vi "Spatial Dual Decode Packet 20 (SubVI).vi"(0 "Packet 20 Bytes In":u8[](array[numeric]), 9 "String Precision":i16) -> (2 "Packet 20 Decoded Data Cluster":T1, 4 "Channel Names":string[](array[string])=["Unix TS", "uS", "Latitude", "Longitude", "Height (m)", "Vel N (m/s)", "Vel E (m/s)", "Vel D (m/s)", "G force (g)", "Pitch (deg)", "Roll (deg)", "Heading (deg)", "Body Acc X (m/s/s)", "Body Acc Y (m/s/s)", "Body Acc Z (m/s/s)", "Angular Vel X (rad/s)", "Angular Vel Y (rad/s)", "Angular Vel Z (rad/s)"], 6 "Data":string[](array[string]), 10 "Channel Units":string[](array[string])=["Unix TS", "uS", "Latitude", "Longitude", "Height (m)", "Vel N (m/s)", "Vel E (m/s)", "Vel D (m/s)", "G force (g)", "Pitch (deg)", "Roll (deg)", "Heading (deg)", "Body Acc X (m/s/s)", "Body Acc Y (m/s/s)", "Body Acc Z (m/s/s)", "Angular Vel X (rad/s)", "Angular Vel Y (rad/s)", "Angular Vel Z (rad/s)"], 14 "Unix Timestamp":u64, 15 "Data Types":string[](array[string])=["seconds", "uS", "deg", "deg", "m", "m/s", "m/s", "m/s", "g", "deg", "deg", "deg", "m/s/s", "m/s/s", "m/s/s", "rad/sec", "rad/sec", "rad/sec"])   [LabVIEW 2019, in "SpatialDual_Parsers.lvlib"]
uses:
  SpatialDual_Parsers.lvlib
  Globals and Definitions/RT Globals RD v1.0.vi
panel:
  out "uS Period":u32
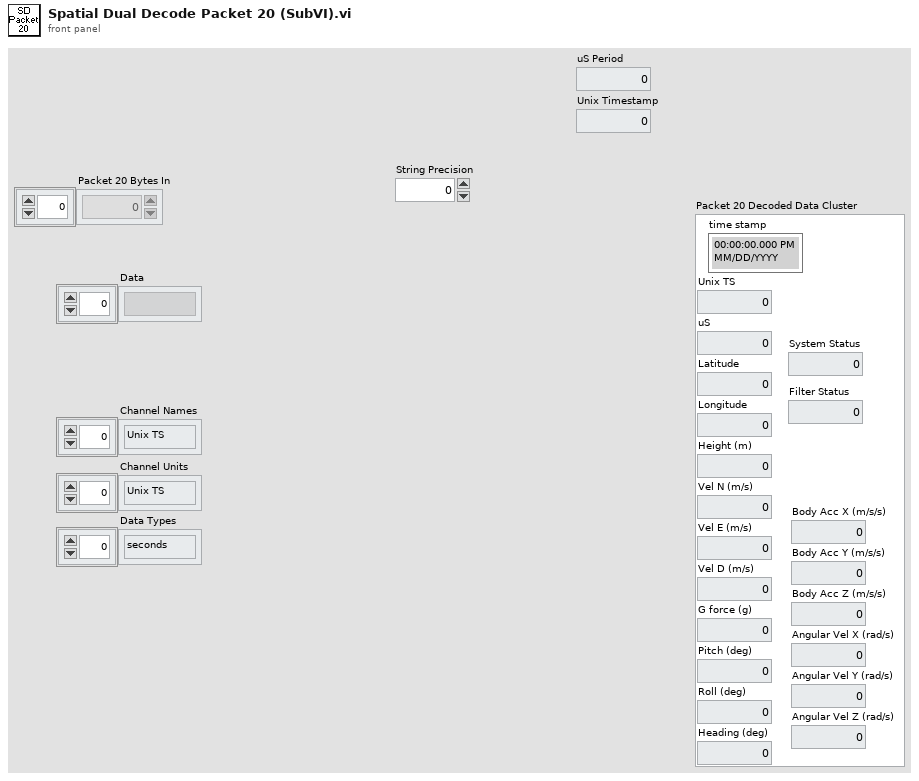
[diagram p1: front panel]
types:
  T1 = cluster{"time stamp":timestamp, "Unix TS":u32, "uS":u32, "Latitude":dbl, "Longitude":dbl, "Height (m)":dbl, "Vel N (m/s)":sgl, "Vel E (m/s)":sgl, "Vel D (m/s)":sgl, "G force (g)":sgl, "Pitch (deg)":sgl, "Roll (deg)":sgl, "Heading (deg)":sgl, "Body Acc X (m/s/s)":sgl, "Body Acc Y (m/s/s)":sgl, "Body Acc Z (m/s/s)":sgl, "Angular Vel X (rad/s)":sgl, "Angular Vel Y (rad/s)":sgl, "Angular Vel Z (rad/s)":sgl, "Filter Status":u16, "System Status":u16}
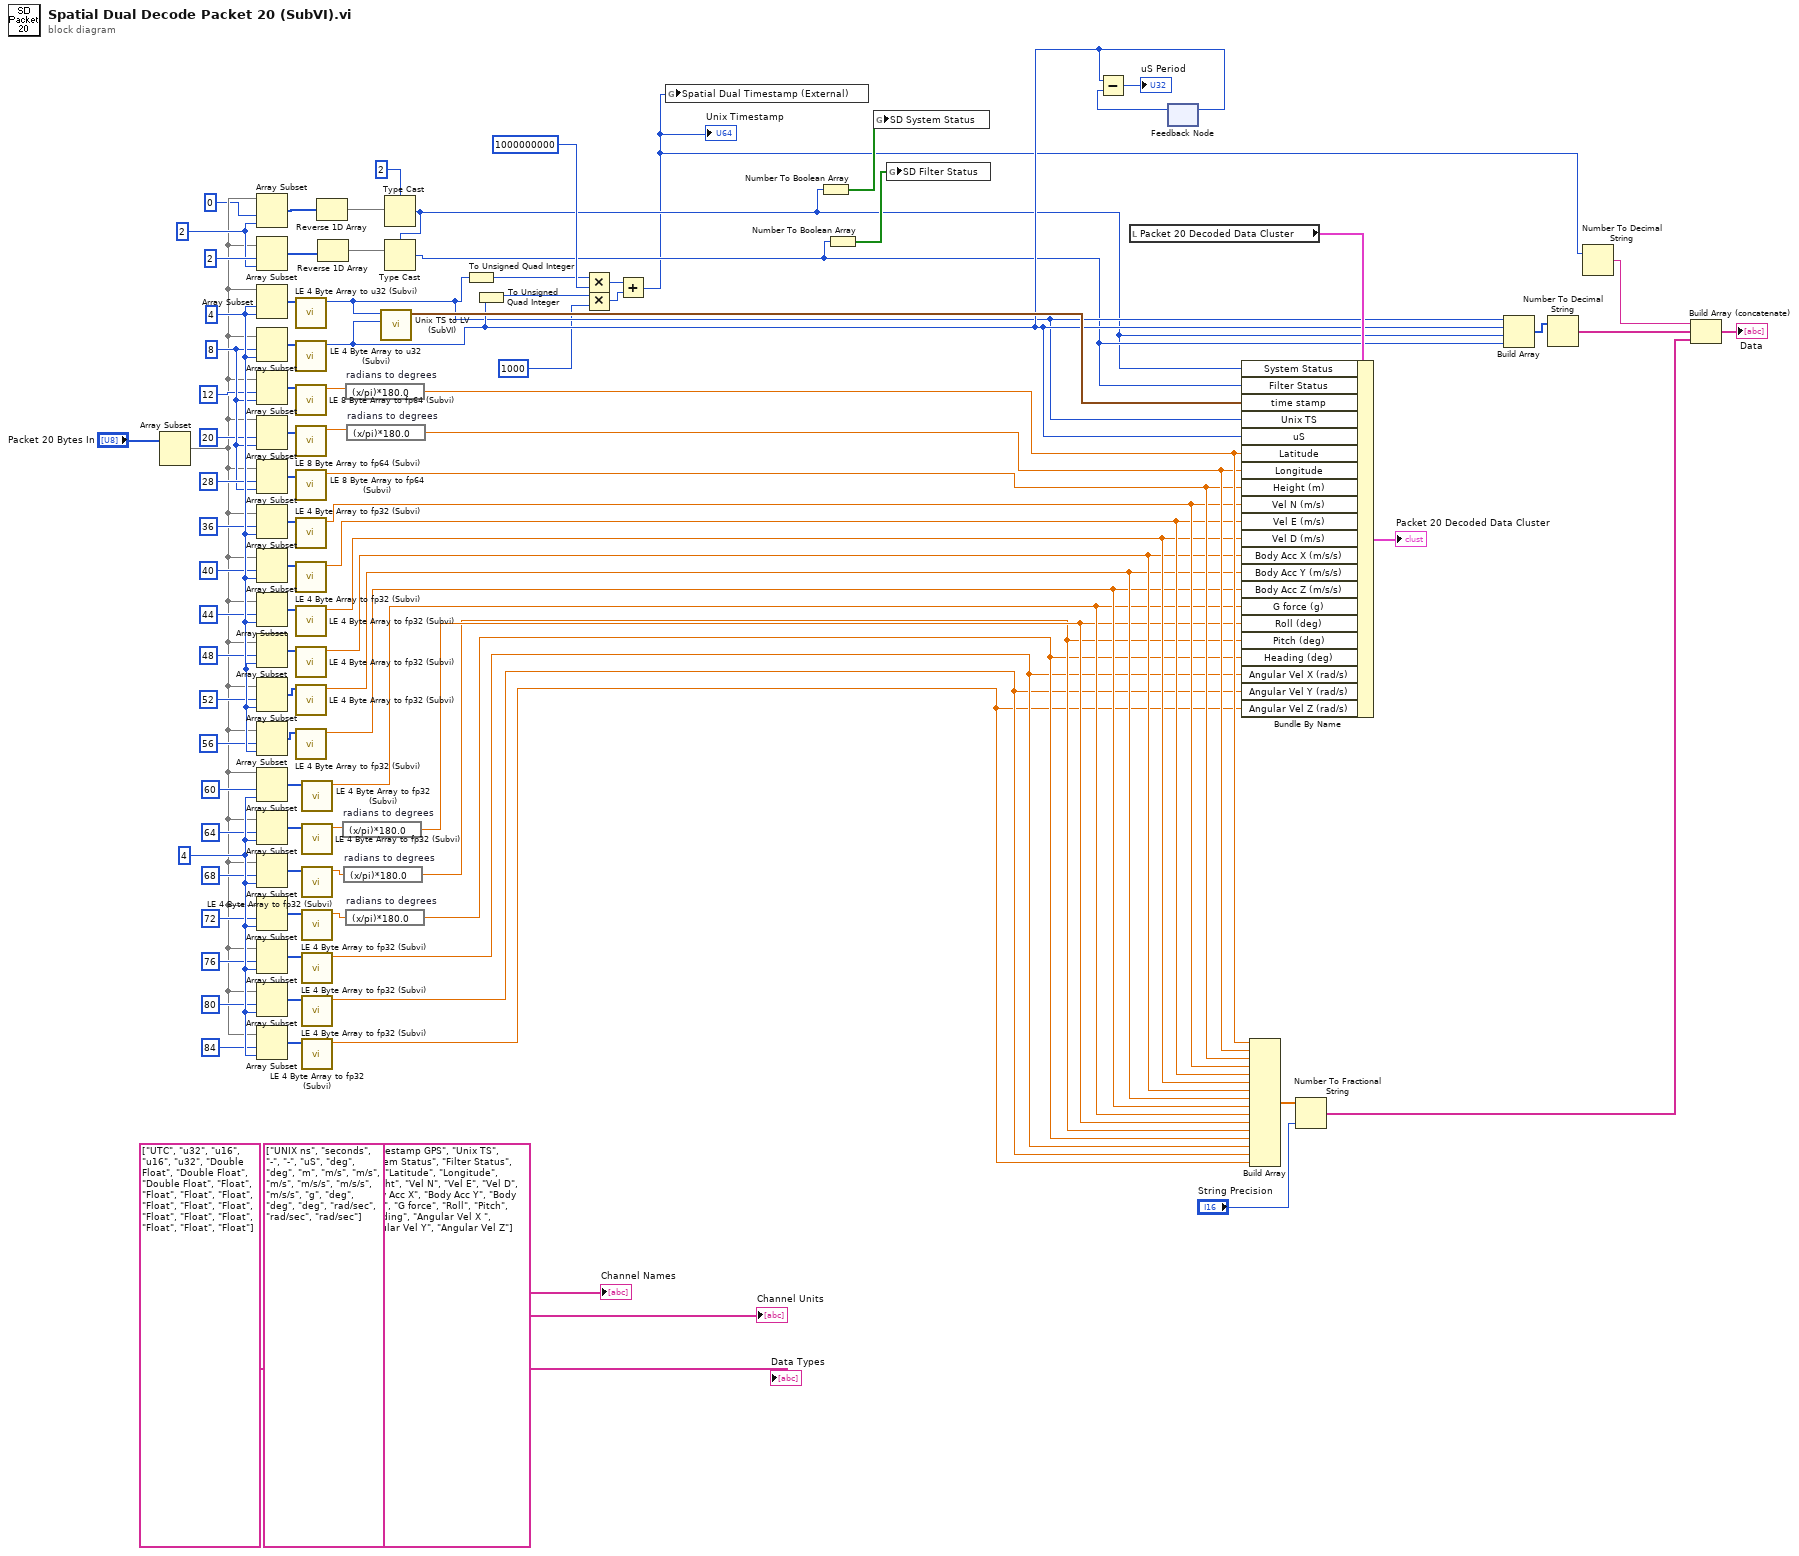
[diagram p0: block diagram]
diagram:
  w26 = 2 ("index")
  w86 = 4 ("index")
  w63 = 8 ("index")
  w77 = 4 ("index")
  n1 = Array Subset(array="Packet 20 Bytes In") -> (w25:u8[])  [unwired: 2 in]
  n2 = Array Subset(array=w25, index=0, length=w26) -> (w18:u8[])
  n3 = Array Subset(array=w25, index=2, length=w26) -> (w21:u8[])
  n4 = Array Subset(array=w25, index=w77, length=w77) -> (w54:u8[])
  n5 = Array Subset(array=w25, index=w63, length=w77) -> (w55:u8[])
  n6 = Array Subset(array=w25, index=12, length=w63) -> (w57:u8[])
  n7 = Array Subset(array=w25, index=20, length=w63) -> (w61:u8[])
  n8 = Array Subset(array=w25, index=28, length=w63) -> (w62:u8[])
  n9 = Array Subset(array=w25, index=36, length=w77) -> (w66:u8[])
  n10 = Array Subset(array=w25, index=40, length=w77) -> (w69:u8[])
  n11 = Array Subset(array=w25, index=44, length=w77) -> (w70:u8[])
  n12 = Array Subset(array=w25, index=48, length=w77) -> (w72:u8[])
  n13 = Array Subset(array=w25, index=52, length=w77) -> (w75:u8[])
  n14 = Array Subset(array=w25, index=56, length=w77) -> (w76:u8[])
  n15 = Array Subset(array=w25, index=60, length=w86) -> (w87:u8[])
  n16 = Array Subset(array=w25, index=64, length=w86) -> (w88:u8[])
  n17 = Array Subset(array=w25, index=68, length=w86) -> (w89:u8[])
  n18 = Array Subset(array=w25, index=72, length=w86) -> (w90:u8[])
  n19 = Array Subset(array=w25, index=76, length=w86) -> (w91:u8[])
  n20 = Array Subset(array=w25, index=80, length=w86) -> (w92:u8[])
  n21 = Array Subset(array=w25, index=84, length=w86) -> (w93:u8[])
  n22 = call "LE 4 Byte Array to u32 (Subvi).vi"("4 Bytes in"=w54) -> ("u32 Out"=w13:u32)  [unwired: 8 in]
  n23 = call "LE 4 Byte Array to u32 (Subvi).vi"("4 Bytes in"=w55) -> ("u32 Out"=w14:u32)  [unwired: 8 in]
  n24 = call "LE 8 Byte Array to fp64 (Subvi).vi"("8 Bytes in"=w57) -> ("fp64 Out"=w58:dbl)  [unwired: 8 in]
  n25 = call "LE 8 Byte Array to fp64 (Subvi).vi"("8 Bytes in"=w61) -> ("fp64 Out"=w60:dbl)  [unwired: 8 in]
  n26 = call "LE 8 Byte Array to fp64 (Subvi).vi"("8 Bytes in"=w62) -> ("fp64 Out"=w42:dbl)  [unwired: 8 in]
  n27 = call "LE 4 Byte Array to fp32 (Subvi).vi"("4 Bytes in"=w66) -> ("fp32 Out"=w41:sgl)  [unwired: 8 in]
  n28 = call "LE 4 Byte Array to fp32 (Subvi).vi"("4 Bytes in"=w69) -> ("fp32 Out"=w40:sgl)  [unwired: 8 in]
  n29 = call "LE 4 Byte Array to fp32 (Subvi).vi"("4 Bytes in"=w70) -> ("fp32 Out"=w39:sgl)  [unwired: 8 in]
  n30 = call "LE 4 Byte Array to fp32 (Subvi).vi"("4 Bytes in"=w72) -> ("fp32 Out"=w38:sgl)  [unwired: 8 in]
  n31 = call "LE 4 Byte Array to fp32 (Subvi).vi"("4 Bytes in"=w75) -> ("fp32 Out"=w37:sgl)  [unwired: 8 in]
  n32 = call "LE 4 Byte Array to fp32 (Subvi).vi"("4 Bytes in"=w76) -> ("fp32 Out"=w36:sgl)  [unwired: 8 in]
  n33 = call "LE 4 Byte Array to fp32 (Subvi).vi"("4 Bytes in"=w87) -> ("fp32 Out"=w35:sgl)  [unwired: 8 in]
  n34 = call "LE 4 Byte Array to fp32 (Subvi).vi"("4 Bytes in"=w88) -> ("fp32 Out"=w94:sgl)  [unwired: 8 in]
  n35 = call "LE 4 Byte Array to fp32 (Subvi).vi"("4 Bytes in"=w89) -> ("fp32 Out"=w95:sgl)  [unwired: 8 in]
  n36 = call "LE 4 Byte Array to fp32 (Subvi).vi"("4 Bytes in"=w90) -> ("fp32 Out"=w96:sgl)  [unwired: 8 in]
  n37 = call "LE 4 Byte Array to fp32 (Subvi).vi"("4 Bytes in"=w91) -> ("fp32 Out"=w31:sgl)  [unwired: 8 in]
  n38 = call "LE 4 Byte Array to fp32 (Subvi).vi"("4 Bytes in"=w92) -> ("fp32 Out"=w30:sgl)  [unwired: 8 in]
  n39 = call "LE 4 Byte Array to fp32 (Subvi).vi"("4 Bytes in"=w93) -> ("fp32 Out"=w29:sgl)  [unwired: 8 in]
  n40 = Reverse 1D Array(array=w18) -> (reversed array=w19:u8[])
  n41 = Reverse 1D Array(array=w21) -> (reversed array=w20:u8[])
  n42 = expression code="(x/pi)*180.0" "radians to degrees"(w94) -> (w34:sgl)
  n43 = expression code="(x/pi)*180.0" "radians to degrees"(w95) -> (w33:sgl)
  n44 = expression code="(x/pi)*180.0" "radians to degrees"(w58) -> (w44:dbl)
  n45 = expression code="(x/pi)*180.0" "radians to degrees"(w96) -> (w32:sgl)
  n46 = expression code="(x/pi)*180.0" "radians to degrees"(w60) -> (w43:dbl)
  n47 = call "Unix TS to LV (SubVI).vi"("mS"=w14, "Unix Time In (s)"=w13) -> ("Labview Time"=w45:timestamp)  [unwired: 9 in]
  n48 = Type Cast(type=u16 2 ("index"), x=w19) -> (*(type *) &x=w5:u16)
  n49 = Type Cast(type=w5, x=w20) -> (*(type *) &x=w8:u16)
  n50 = To Unsigned Quad Integer(1:w13) -> (0:w4:u64)
  n51 = To Unsigned Quad Integer(1:w14) -> (0:w12:u64)
  n52 = Multiply(x=w4, y=u64 1000000000 ("sec")) -> (x*y=w10:u64)
  n53 = Multiply(x=w12, y=u64 1000 ("us")) -> (x*y=w9:u64)
  n54 = Add(x=w10, y=w9) -> (x+y=w3:u64)
  "Unix Timestamp" <- w3
  n55 = global write "RT Globals RD v1.0.vi" "Spatial Dual Timestamp (External)"(w3) -> ()
  n56 = Number To Boolean Array(number=w5) -> (Boolean array=w6:bool[])
  n57 = Number To Boolean Array(number=w8) -> (Boolean array=w7:bool[])
  n58 = global write "RT Globals RD v1.0.vi" "SD System Status"(w6) -> ()
  n59 = global write "RT Globals RD v1.0.vi" "SD Filter Status"(w7) -> ()
  n60 = local read "Packet 20 Decoded Data Cluster"() -> (w22:T1)
  n61 = feedback-in #1(w14) -> ()
  n62 = feedback #1() -> (w17:u32)  [unwired: 1 in]
  n63 = Subtract(x=w14, y=w17) -> (x-y=→"uS Period":u32)
  n64 = Bundle By Name(cluster=w22, "System Status"=w5, "Filter Status"=w8, "time stamp"=w45, "Unix TS"=w13, "uS"=w14, "Latitude"=w44, "Longitude"=w43, "Height (m)"=w42, "Vel N (m/s)"=w41, "Vel E (m/s)"=w40, "Vel D (m/s)"=w39, "Body Acc X (m/s/s)"=w38, "Body Acc Y (m/s/s)"=w37, "Body Acc Z (m/s/s)"=w36, "G force (g)"=w35, "Roll (deg)"=w34, "Pitch (deg)"=w33, "Heading (deg)"=w32, "Angular Vel X (rad/s)"=w31, "Angular Vel Y (rad/s)"=w30, "Angular Vel Z (rad/s)"=w29) -> (→"Packet 20 Decoded Data Cluster":T1)
  n65 = Build Array(w44, w43, w42, w41, w40, w39, w38, w37, w36, w35, w34, w33, w32, w31, w30, w29) -> (w28:dbl[])
  n66 = Number To Fractional String(number=w28, precision (6)="String Precision") -> (F-format string=w49:string[])  [unwired: 2 in]
  n67 = Build Array(w13, w14, w5, w8) -> (w48:u32[])
  n68 = Number To Decimal String(number=w48) -> (decimal integer string=w47:string[])  [unwired: 1 in]
  n69 = Number To Decimal String(number=w3) -> (decimal integer string=w2:string)  [unwired: 1 in]
  n70 = Build Array (concatenate)(w2, w47, w49) -> (→"Data":string[])
  "Channel Names" <- string[] ["Timestamp GPS", "Unix TS", "System Status", "Filter Status", "uS", "Latitude", "Longitude", "Height", "Vel N", "Vel E", "Vel D", "Body Acc X", "Body Acc Y", "Body Acc Z", "G force", "Roll", "Pitch", "Heading", "Angular Vel X ", "Angular Vel Y", "Angular Vel Z"] ("Array")
  "Channel Units" <- string[] ["UNIX ns", "seconds", "-", "-", "uS", "deg", "deg", "m", "m/s", "m/s", "m/s", "m/s/s", "m/s/s", "m/s/s", "g", "deg", "deg", "deg", "rad/sec", "rad/sec", "rad/sec"] ("Array")
  "Data Types" <- string[] ["UTC", "u32", "u16", "u16", "u32", "Double Float", "Double Float", "Double Float", "Float", "Float", "Float", "Float", "Float", "Float", "Float", "Float", "Float", "Float", "Float", "Float", "Float"] ("Array")
